vi "serial robot1.vi"(0 "Numeric":dbl, 1 "Numeric 2":dbl, 2 "Numeric 3":dbl, 3 "Numeric 4":dbl) -> ()   [LabVIEW 2010]
doc: "The Basic Serial Read and Write example performs a Serial Port Read, a Serial Port Write, or a combination of these actions. The user selects the actions (read or write) on the front panel. If both are selected, the VI will write the data first, read data, and then close the VISA session that is opened to the port. This VI will wait until the specified number of bytes is received at the port or until a termination character is read.\n\nINSTRUCTIONS:\n1) Select the serial resource and configuration parameters (baud rate, data bits, parity, stop bits, flow control).\n2) Select the operations to be performed. \n3) Connect the serial port to your device. If no device is available, perform a loopback test by doing one of the following. Short pins 2 and 3 on a RS-232 cable or short pin 4 to pin 8 and pin 5 to pin 9 on a RS-485/422 cable. \n4) Run the VI to see the data read. (The \"read string\" will match the \"string to write\" if a loopback test was performed.)\n\nNote: The parameters set for the serial port must match the parameters of the connected instrument or device. In this example, the bytes to read parameter specifies the number of bytes that the serial port reads. If there were more bytes at the port than the number specified in bytes to read, those bytes would not be read. Also, if you specify to read more bytes than the number of bytes actually read, you might receive a timeout error message.\n\nOn the block diagram, the Configure Serial Port VI sets the configuration parameters. The front panel displays the controls used to configure the basic parameters, such as baud rate, data bits, and parity. Constants configure the other parameters the user probably does not need set. After the VISA Configure Serial Port VI opens the VISA session and configures the port, the VI passes the VISA resource name to other VIs that perform operations on that VISA resource. The VISA Write function sends a command to the serial device and the VISA Read function returns data based on the command. The VISA Close function then closes the reference to the serial device. It is important to close the reference; otherwise communication through with that port through protocols other than VISA might not be possible."
uses:
  <vilib>/Instr/_visa.llb/VISA Configure Serial Port (Instr).vi
panel:
  out "String":string="mo4"
  out "concatenated string 4":string
  out "concatenated string 3":string
  out "concatenated string 2":string
  out "substring 9":string
  out "substring 8":string
  out "substring 2":string
  out "substring":string
  out "Numeric 11":i32
  out "Numeric 10":i32
  out "Numeric 9":i32
  in  "flow control 2":u16(ring) items=["None"=0, "XON/XOFF"=1, "RTS/CTS"=2, "DTR/DSR"=4]
  in  "stop bits 2":u16(ring)=10 items=["1.0"=10, "1.5"=15, "2.0"=20]
  in  "parity 2":u16(ring) items=["None", "Odd", "Even", "Mark", "Space"]
  in  "data bits 2":u16=8 min=5 max=8 step=1
  in  "VISA resource name 2":refnum<visa-resource-name>="COM1"
  out "Numeric 8":i32
  out "substring 4":string
  out "concatenated string":string
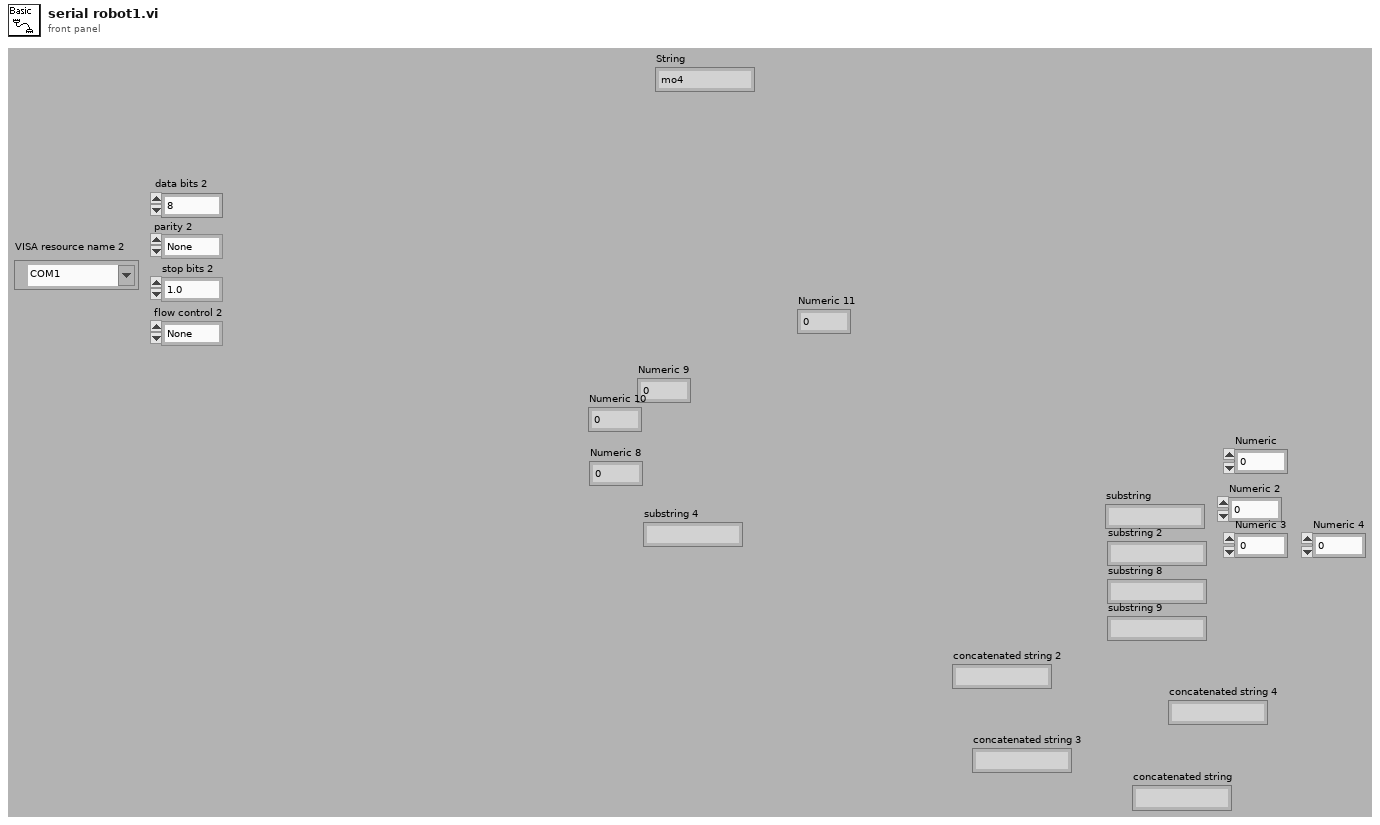
[diagram p1: front panel]
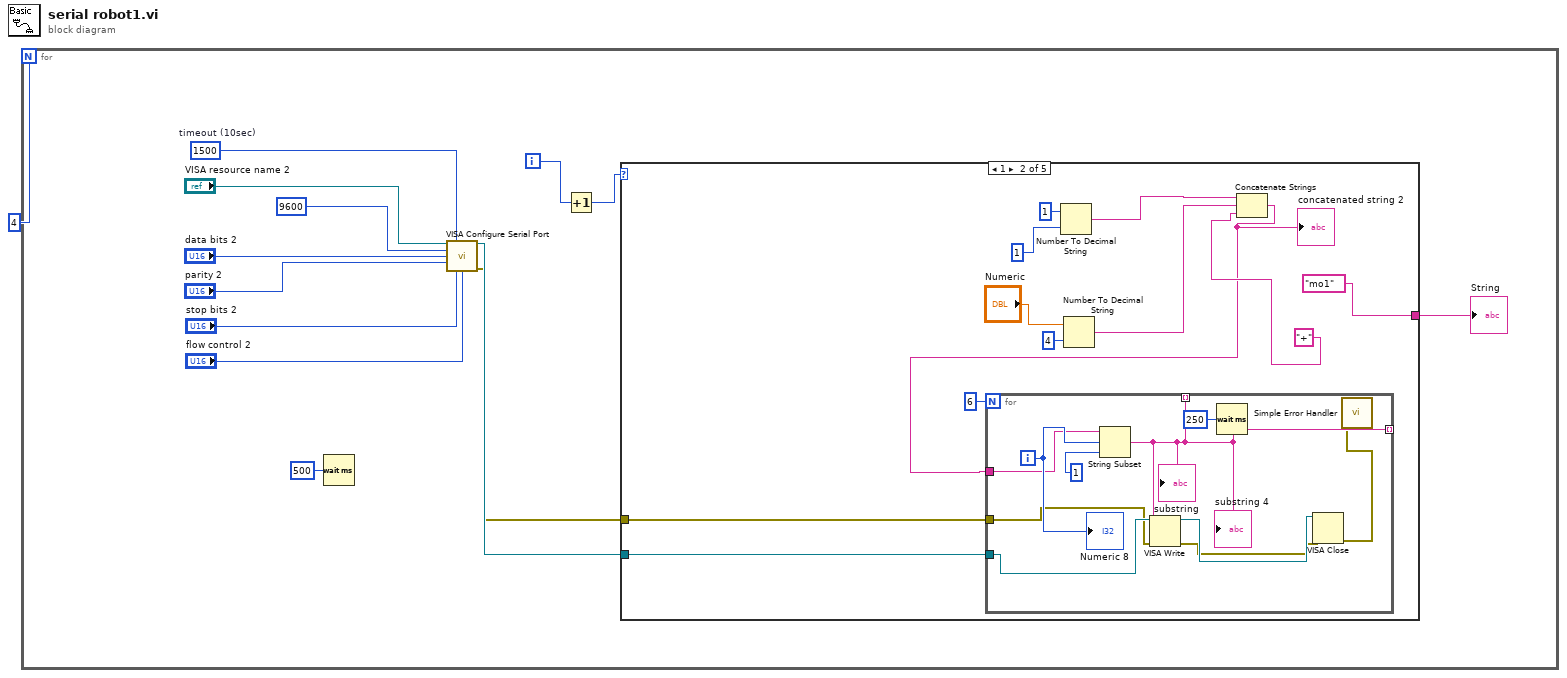
[diagram p0: block diagram]
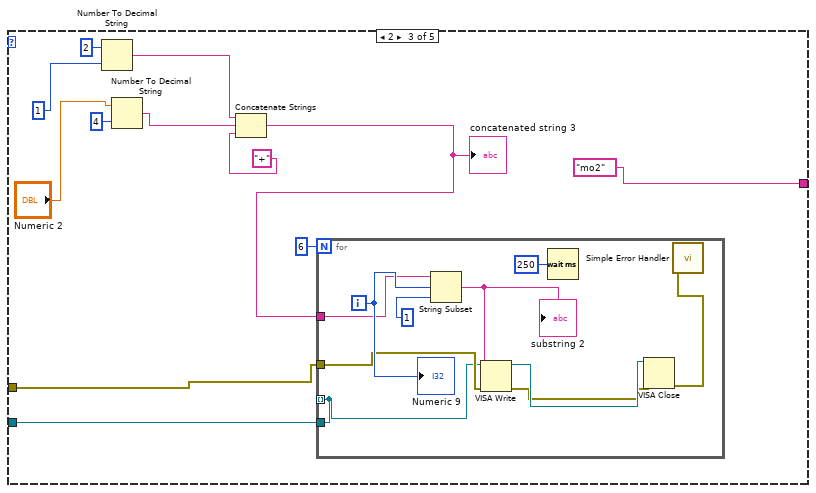
[diagram p3: hidden frame]
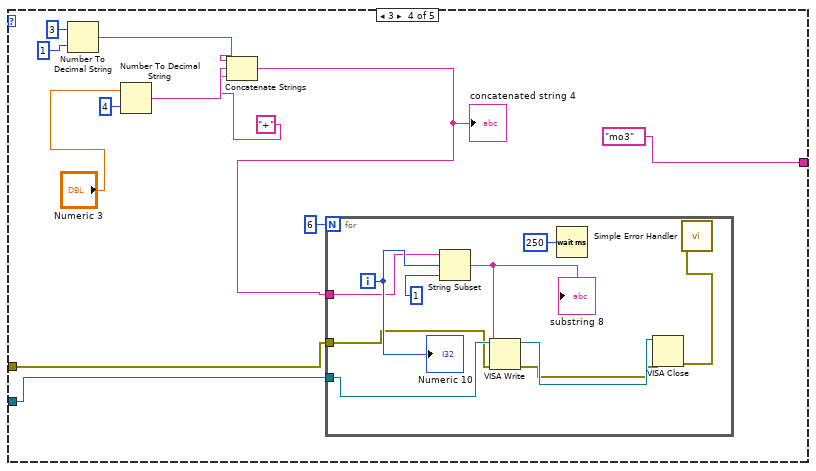
[diagram p4: hidden frame]
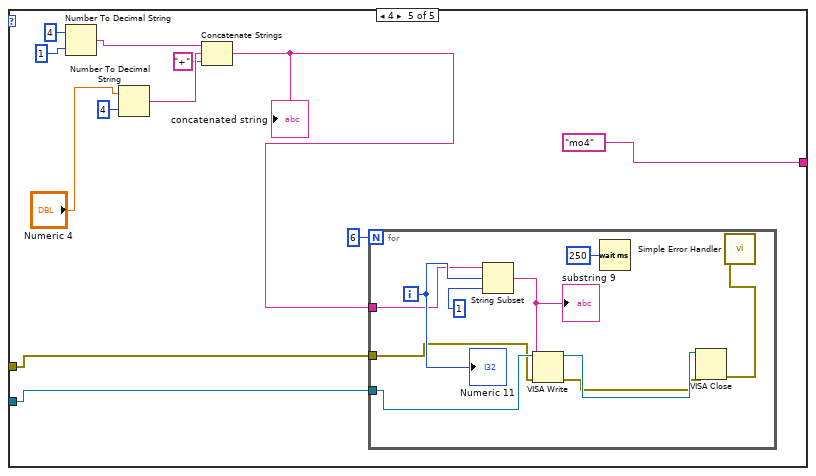
[diagram p5: hidden frame]
diagram:
  n1 = for {
    N: 4 -> [_]
    i -> [w4]
    w10 = u32 1500  # timeout (10sec)
    n2 = Wait (ms)(milliseconds to wait=u32 500) -> ()  [unwired: 1 out]
    n3 = call-poly "VISA Configure Serial Port"("VISA resource name"="VISA resource name 2", "timeout (10sec)"=w10, "baud rate (9600)"=u32 9600 ("baud rate"), "data bits (8)"="data bits 2", "parity (0:none)"="parity 2", "stop bits (10: 1 bit)"="stop bits 2", "flow control (0:none)"="flow control 2") -> ("VISA resource name out"=w7:refnum<visa-resource-name>, "error out"=w6:errorcluster)  [unwired: 2 in, 5 out]
    n4 = Increment(x=w4) -> (x+1=w3:i32)
    n5 = case shown="1" w3 {
      tunnel: w7 -> [_ w19 w40 w62 w83]
      tunnel: w6 -> [_ w18 w41 w63 w84]
      tunnel: [_ "mo1" "mo2" "mo3" "mo4"] -> w2
      frame 0, Default {
      }
      frame 1 {
        n6 = Number To Decimal String(number=1, width (-)=i16 1) -> (decimal integer string=w23:string)
        n7 = Number To Decimal String(number="Numeric", width (-)=i16 4) -> (decimal integer string=w22:string)
        n8 = Concatenate Strings(w23, w22, "+" ("string")) -> (w17:string)
        "concatenated string 2" <- w17
        n9 = for {
          N: 6 -> [_]
          tunnel: [w34] -> _ mode=indexing
          tunnel: [w34] -> _ mode=indexing
          tunnel: w19 -> [w28]
          tunnel: w17 -> [w32]
          tunnel: w18 -> [w27]
          i -> [w36]
          n10 = String Subset(string=w32, offset (0)=w36, length (rest)=1 ("length (rest)")) -> (substring=w34:string)
          "substring 4" <- w34
          "substring" <- w34
          n11 = VISA Write(VISA resource name=w28, write buffer=w34, error in (no error)=w27) -> (VISA resource name out=w31:refnum<visa-resource-name>, error out=w30:errorcluster)  [unwired: 1 out]
          n12 = Wait (ms)(milliseconds to wait=u32 250) -> ()  [unwired: 1 out]
          n13 = VISA Close(VISA resource name=w31, error in (no error)=w30) -> (error out=w33:errorcluster)
          n14 = call <vilib>:"Simple Error Handler.vi"("error in (no error)"=w33) -> ()  [unwired: 1 in, 8 out]
          "Numeric 8" <- w36
        }
      }
      frame 2 {
        n15 = Number To Decimal String(number=2, width (-)=i16 1) -> (decimal integer string=w44:string)
        n16 = Number To Decimal String(number="Numeric 2", width (-)=i16 4) -> (decimal integer string=w45:string)
        n17 = Concatenate Strings(w44, w45, "+" ("string")) -> (w39:string)
        "concatenated string 3" <- w39
        n18 = for {
          N: 6 -> [_]
          tunnel: [w49] -> _ mode=indexing
          tunnel: w39 -> [w54]
          tunnel: w41 -> [w50]
          tunnel: w40 -> [w49]
          i -> [w58]
          n19 = String Subset(string=w54, offset (0)=w58, length (rest)=1 ("length (rest)")) -> (substring=w56:string)
          "substring 2" <- w56
          n20 = VISA Write(VISA resource name=w49, write buffer=w56, error in (no error)=w50) -> (VISA resource name out=w53:refnum<visa-resource-name>, error out=w52:errorcluster)  [unwired: 1 out]
          n21 = Wait (ms)(milliseconds to wait=u32 250) -> ()  [unwired: 1 out]
          n22 = VISA Close(VISA resource name=w53, error in (no error)=w52) -> (error out=w55:errorcluster)
          n23 = call <vilib>:"Simple Error Handler.vi"("error in (no error)"=w55) -> ()  [unwired: 1 in, 8 out]
          "Numeric 9" <- w58
        }
      }
      frame 3 {
        n24 = Number To Decimal String(number=3, width (-)=i16 1) -> (decimal integer string=w67:string)
        n25 = Number To Decimal String(number="Numeric 3", width (-)=i16 4) -> (decimal integer string=w66:string)
        n26 = Concatenate Strings(w67, w66, "+" ("string")) -> (w61:string)
        "concatenated string 4" <- w61
        n27 = for {
          N: 6 -> [_]
          tunnel: w62 -> [w72]
          tunnel: w61 -> [w76]
          tunnel: w63 -> [w71]
          i -> [w80]
          n28 = String Subset(string=w76, offset (0)=w80, length (rest)=1 ("length (rest)")) -> (substring=w78:string)
          "substring 8" <- w78
          n29 = VISA Write(VISA resource name=w72, write buffer=w78, error in (no error)=w71) -> (VISA resource name out=w75:refnum<visa-resource-name>, error out=w74:errorcluster)  [unwired: 1 out]
          n30 = Wait (ms)(milliseconds to wait=u32 250) -> ()  [unwired: 1 out]
          n31 = VISA Close(VISA resource name=w75, error in (no error)=w74) -> (error out=w77:errorcluster)
          n32 = call <vilib>:"Simple Error Handler.vi"("error in (no error)"=w77) -> ()  [unwired: 1 in, 8 out]
          "Numeric 10" <- w80
        }
      }
      frame 4 {
        n33 = Number To Decimal String(number=4, width (-)=i16 1) -> (decimal integer string=w88:string)
        n34 = Number To Decimal String(number="Numeric 4", width (-)=i16 4) -> (decimal integer string=w89:string)
        n35 = Concatenate Strings(w88, w89, "+" ("string")) -> (w85:string)
        "concatenated string" <- w85
        n36 = for {
          N: 6 -> [_]
          tunnel: w83 -> [w95]
          tunnel: w85 -> [w99]
          tunnel: w84 -> [w94]
          i -> [w102]
          n37 = String Subset(string=w99, offset (0)=w102, length (rest)=1 ("length (rest)")) -> (substring=w93:string)
          "substring 9" <- w93
          n38 = VISA Write(VISA resource name=w95, write buffer=w93, error in (no error)=w94) -> (VISA resource name out=w98:refnum<visa-resource-name>, error out=w97:errorcluster)  [unwired: 1 out]
          n39 = Wait (ms)(milliseconds to wait=u32 250) -> ()  [unwired: 1 out]
          n40 = VISA Close(VISA resource name=w98, error in (no error)=w97) -> (error out=w100:errorcluster)
          n41 = call <vilib>:"Simple Error Handler.vi"("error in (no error)"=w100) -> ()  [unwired: 1 in, 8 out]
          "Numeric 11" <- w102
        }
      }
    }
    "String" <- w2
  }
